vi "Configure Trigger (Window).vi"(0 "VISA resource name":refnum<visa-resource-name>, 1 "Trigger Point (0: Boundary)":i32(ring) items=["Boundary", "Timeout"], 5 "Trigger Source (1: Channel1)":i32(ring)=1 items=["Channel1"=1, "Channel2"=2, "Channel3"=3, "Channel4"=4], 7 "Condition (0: Enter)":i32(ring) items=["Enter", "Exit", "Insider (Greater Than)", "Insider (Low Than)", "Outside (Greater Than)", "Outside (Lower Than)"], 9 "Limit Time (1E-9 s)":dbl=1e-09, 11 "error in (no error)":errorcluster) -> (4 "VISA resource name out":refnum<visa-resource-name>, 15 "error out":errorcluster)   [LabVIEW 2020, in "Agilent 90000 Series.lvlib"]
doc: "Configures window trigger parameters."
uses:
  Agilent 90000 Series.lvlib
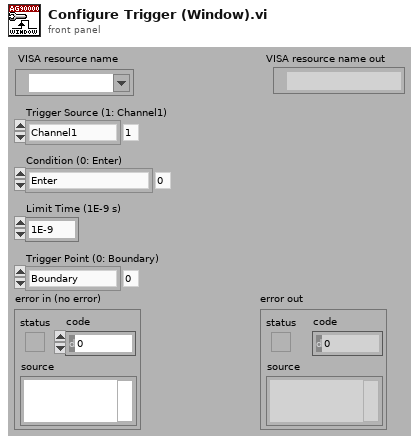
[diagram p1: front panel]
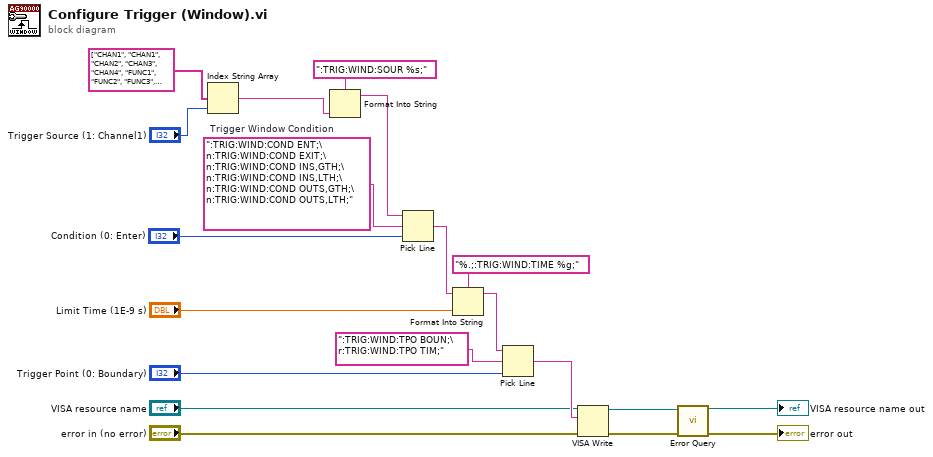
[diagram p0: block diagram]
diagram:
  w3 = ":TRIG:WIND:COND ENT;\n:TRIG:WIND:COND EXIT;\n:TRIG:WIND:COND INS,GTH;\n:TRIG:WIND:COND INS,LTH;\n:TRIG:WIND:COND OUTS,GTH;\n:TRIG:WIND:COND OUTS,LTH;"  # Trigger Window Condition
  n1 = Index String Array(1:"Trigger Source (1: Channel1)", 2:string[] ["CHAN1", "CHAN1", "CHAN2", "CHAN3", "CHAN4", "FUNC1", "FUNC2", "FUNC3", "FUNC4", "WMEM1", "WMEM2", "WMEM3", "WMEM4", "AUX", "LINE", ""]) -> (0:w5:string)  [unwired: 1 out]
  n2 = Format Into String(format string=":TRIG:WIND:SOUR %s;", w5) -> (resulting string=w2:string)  [unwired: 2 in, 1 out]
  n3 = Pick Line(string ("")=w2, multi-line string=w3, line index="Condition (0: Enter)") -> (output string=w1:string)
  n4 = Format Into String(format string="%.;:TRIG:WIND:TIME %g;", initial string=w1, "Limit Time (1E-9 s)") -> (resulting string=w18:string)  [unwired: 1 in, 1 out]
  n5 = Pick Line(string ("")=w18, multi-line string=":TRIG:WIND:TPO BOUN;\r:TRIG:WIND:TPO TIM;", line index="Trigger Point (0: Boundary)") -> (output string=w15:string)
  n6 = VISA Write(VISA resource name="VISA resource name", write buffer=w15, error in (no error)="error in (no error)") -> (VISA resource name out=w12:refnum<visa-resource-name>, error out=w11:errorcluster)  [unwired: 1 out]
  n7 = call "Error Query.vi"("error in (no error)"=w11, "VISA resource name"=w12) -> ("error out"=→"error out":errorcluster, "VISA resource name out"=→"VISA resource name out":refnum<visa-resource-name>)  [unwired: 8 out]
